vi "NanotecSMCPDDriver.application example1.vi"() -> ()   [LabVIEW 2014, in "NanotecSMCPDDriver.lvlib"]
doc: "an application example for using the instrument driver"
uses:
  NanotecSMCPDDriver.lvlib
  Action-Status/NanotecSMCPDDriver.status type.ctl
panel:
  in  "findReference":bool
  in  "abortMove":bool
  in  "moveRelative":bool
  in  "moveAbsolute":bool
  in  "Exit":bool
  in  "position [uSteps]":i32
  out "actPosition [usteps]":i32
  out "actStatus":T1
  out "Instrument Firmware Revision":string
  out "Instrument Driver Revision":string
  out "error out":errorcluster
  in  "Reset (True)":bool
  in  "ID Query (True)":bool
  in  "contollerID":i32=1
  in  "VISA resource name":refnum<visa-resource-name>="COM3"
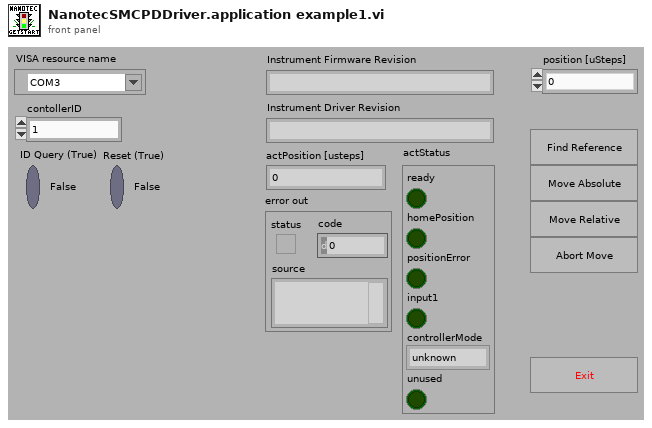
[diagram p1: front panel]
types:
  T1 = typedef "NanotecSMCPDDriver.lvlib/NanotecSMCPDDriver.status type.ctl" = cluster{"ready":bool, "homePosition":bool, "positionError":bool, "input1":bool, "controllerMode":enum16{"unknown", "position", "speed", "flagPosition", "clockDirection", "analog", "joystick", "unused"}, "unused":bool}
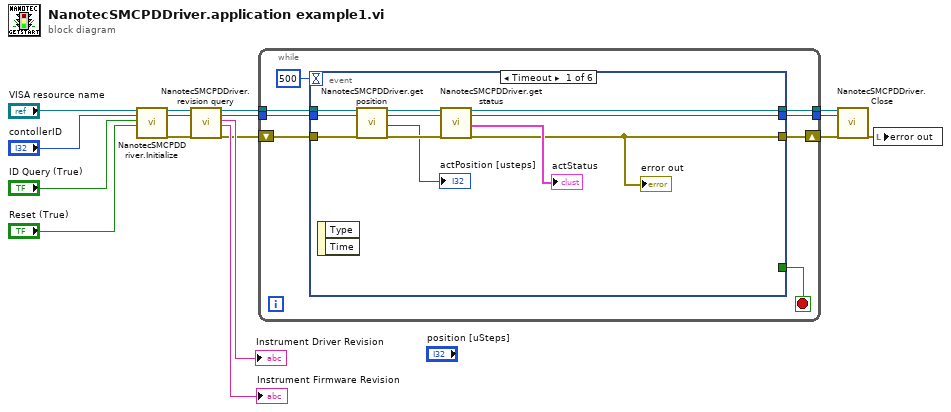
[diagram p0: block diagram]
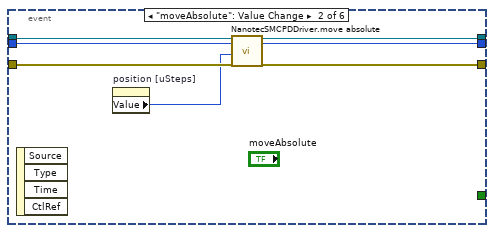
[diagram p2: hidden frame]
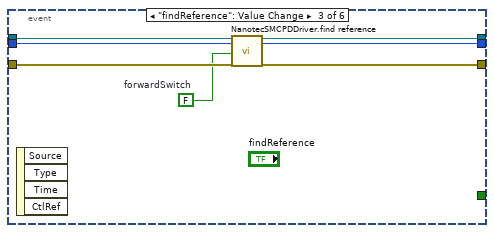
[diagram p3: hidden frame]
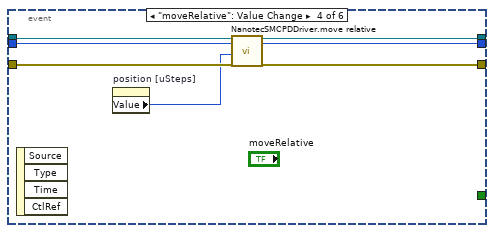
[diagram p4: hidden frame]
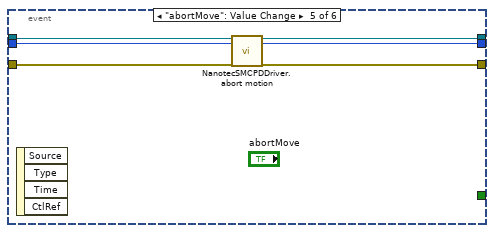
[diagram p5: hidden frame]
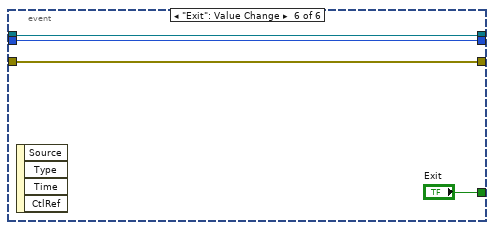
[diagram p6: hidden frame]
diagram:
  n1 = call "NanotecSMCPDDriver.Initialize.vi"("VISA resource name"="VISA resource name", "contollerID"="contollerID", "ID Query (True)"="ID Query (True)", "Reset (True)"="Reset (True)") -> ("VISA resource name out"=w10:refnum<visa-resource-name>, "contollerID out"=w9:i32, "error out"=w8:errorcluster)  [unwired: 13 in]
  n2 = call "NanotecSMCPDDriver.revision query.vi"("VISA resource name"=w10, "contollerID"=w9, "error in (no error)"=w8) -> ("VISA resource name out"=w7:refnum<visa-resource-name>, "contollerID out"=w3:i32, "Instrument Driver Revision"=→"Instrument Driver Revision":string, "Instrument Firmware Revision"=→"Instrument Firmware Revision":string, "error out"=w5:errorcluster)  [unwired: 12 in]
  n3 = while {
    tunnel: w7 -> [w24]
    tunnel: [w22] -> w6
    tunnel: w3 -> [w19]
    tunnel: [w18] -> w2
    shift-right: [w20] -> w4
    shift-left: w5 -> [w21]
    stop <- w23 stop-if-true
    n4 = event shown="[0] Timeout" {
      selector: _ -> [_ _ _ _ _ _]
      dyn-events: _ -> [_ _ _ _ _ _]
      timeout: 500 -> [_ _ _ _ _ _]
      tunnel: w24 -> [w35 w42 w49 w56 w62 w65]
      tunnel: [_ _ _ _ _ "Exit"] -> w23
      tunnel: [w29 w39 w46 w53 w59 w65] -> w22
      tunnel: w21 -> [w33 w40 w47 w54 w60 w64]
      tunnel: [w25 w37 w44 w51 w57 w64] -> w20
      tunnel: w19 -> [w34 w41 w48 w55 w61 w63]
      tunnel: [w28 w38 w45 w52 w58 w63] -> w18
      event Timeout {
        n5 = event-data() -> ()  [unwired: 1 in, 2 out]
        n6 = call "NanotecSMCPDDriver.get position.vi"("VISA resource name"=w35, "contollerID"=w34, "error in (no error)"=w33) -> ("VISA resource name out"=w32:refnum<visa-resource-name>, "contollerID out"=w31:i32, "actPosition [usteps]"=→"actPosition [usteps]":i32, "error out"=w30:errorcluster)  [unwired: 13 in]
        n7 = call "NanotecSMCPDDriver.get status.vi"("VISA resource name"=w32, "contollerID"=w31, "error in (no error)"=w30) -> ("VISA resource name out"=w29:refnum<visa-resource-name>, "contollerID out"=w28:i32, "actStatus"=→"actStatus":T1, "error out"=w25:errorcluster)  [unwired: 13 in]
        "error out" <- w25
      }
      event "moveAbsolute": Value Change {
        n8 = event-data() -> ()  [unwired: 1 in, 4 out]
        n9 = property on="position [uSteps]" class="DigNum (strict)"() -> ("Value"=w36:i32)  [unwired: 2 in, 2 out]
        n10 = call "NanotecSMCPDDriver.move absolute.vi"("VISA resource name"=w42, "contollerID"=w41, "nOfSteps [uSteps]"=w36, "error in (no error)"=w40) -> ("VISA resource name out"=w39:refnum<visa-resource-name>, "contollerID out"=w38:i32, "error out"=w37:errorcluster)  [unwired: 13 in]
      }
      event "findReference": Value Change {
        w43 = FALSE  # forwardSwitch
        n11 = event-data() -> ()  [unwired: 1 in, 4 out]
        n12 = call "NanotecSMCPDDriver.find reference.vi"("VISA resource name"=w49, "contollerID"=w48, "forwardSwitch"=w43, "error in (no error)"=w47) -> ("VISA resource name out"=w46:refnum<visa-resource-name>, "contollerID out"=w45:i32, "error out"=w44:errorcluster)  [unwired: 13 in]
      }
      event "moveRelative": Value Change {
        n13 = event-data() -> ()  [unwired: 1 in, 4 out]
        n14 = property on="position [uSteps]" class="DigNum (strict)"() -> ("Value"=w50:i32)  [unwired: 2 in, 2 out]
        n15 = call "NanotecSMCPDDriver.move relative.vi"("VISA resource name"=w56, "contollerID"=w55, "nOfSteps [uSteps]"=w50, "error in (no error)"=w54) -> ("VISA resource name out"=w53:refnum<visa-resource-name>, "contollerID out"=w52:i32, "error out"=w51:errorcluster)  [unwired: 13 in]
      }
      event "abortMove": Value Change {
        n16 = event-data() -> ()  [unwired: 1 in, 4 out]
        n17 = call "NanotecSMCPDDriver.abort motion.vi"("VISA resource name"=w62, "contollerID"=w61, "error in (no error)"=w60) -> ("VISA resource name out"=w59:refnum<visa-resource-name>, "contollerID out"=w58:i32, "error out"=w57:errorcluster)  [unwired: 14 in]
      }
      event "Exit": Value Change {
        n18 = event-data() -> ()  [unwired: 1 in, 4 out]
      }
    }
  }
  n19 = call "NanotecSMCPDDriver.Close.vi"("VISA resource name"=w6, "contollerID"=w2, "error in (no error)"=w4) -> ("error out"=w1:errorcluster)  [unwired: 16 in]
  n20 = local write "error out"(w1) -> ()
